vi "CRYInsert Data to Listbox Etc.vi"(4 "Type":enum16{"Curves", "Values", "Results", "WFM"}(ring)=enum."Results", 7 "sAction":string, 8 "Waveforms":T2[](array[typedef]) {"Y dB ref" format="%.1f"; "Y axis" items=["Log", "Lin"]; "Y data" items=["dB", "Lin"]; "X data" items=["dB", "Lin"]}, 9 "Results":T3[](array[typedef]) {"Margin" format="%.2f"}, 10 "Values":T1[](array[typedef]) {"Z data" items=["dB", "Lin"]; "X data" items=["dB", "Lin"]; "Y data" items=["dB", "Lin"]; "Z dB ref" format="%.1f"; "Z axis" items=["Log", "Lin"]; "X dB ref" format="%.1f"; "X axis" items=["Log", "Lin"]; "Y axis" items=["Log", "Lin"]; "Y dB ref" format="%.1f"; "Curve"."z" format="%.2f"; "Curve"."y" format="%.2f"; "Curve"."x" format="%.2f"}, 11 "Curves":T1[](array[typedef]) {"Z data" items=["dB", "Lin"]; "X data" items=["dB", "Lin"]; "Y data" items=["dB", "Lin"]; "Z dB ref" format="%.1f"; "Z axis" items=["Log", "Lin"]; "X dB ref" format="%.1f"; "X axis" items=["Log", "Lin"]; "Y axis" items=["Log", "Lin"]; "Y dB ref" format="%.1f"; "Curve"."z" format="%.2f"; "Curve"."y" format="%.2f"; "Curve"."x" format="%.2f"}) -> ()   [LabVIEW 2013]
uses:
  CRYSystem/Typedef Control/CRYData Cluster.ctl
  CRYSystem/Typedef Control/CRYResult Cluster.ctl
  CRYSystem/Typedef Control/CRYWaveform Cluster.ctl
  Global/CRYCurve Library Global.vi
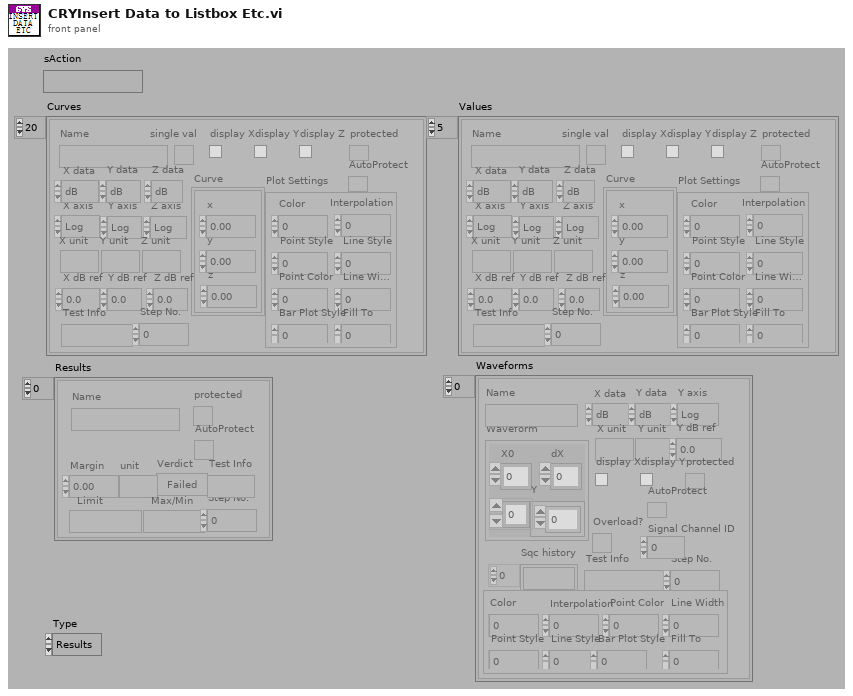
[diagram p1: front panel]
types:
  T1 = typedef "CRYData Cluster.ctl" = cluster{"Name":string, "Curve":cluster{"x":dbl, "y":dbl, "z":dbl}[], "X data":u16, "Y data":u16, "Z data":u16, "X axis":u16, "Y axis":u16, "Z axis":u16, "X unit":string, "Y unit":string, "Z unit":string, "X dB ref":dbl, "Y dB ref":dbl, "Z dB ref":dbl, "single val":bool, "protected":bool, "display X":bool, "display Y":bool, "display Z":bool, "Test Info":string, "Step No.":i32, "Plot Settings":cluster{"Color":u32, "Interpolation":u8, "Point Style":u8, "Line Style":u8, "Point Color":u32, "Line Width":u8, "Bar Plot Style":u8, "Fill To":i16}, "AutoProtect":bool}
  T2 = typedef "CRYWaveform Cluster.ctl" = cluster{"Waveform":cluster{"X0":dbl, "dX":dbl, "Y":sgl[]}, "X data":u16, "Y data":u16, "Y axis":u16, "X unit":string, "Y unit":string, "Y dB ref":dbl, "display Y":bool, "display X":bool, "Overload?":bool, "Test Info":string, "Step No.":i32, "Name":string, "protected":bool, "Sqc history":string[], "Signal Channel ID":i32, "Plot Settings":cluster{"Color":u32, "Interpolation":u8, "Point Style":u8, "Line Style":u8, "Point Color":u32, "Line Width":u8, "Bar Plot Style":u8, "Fill To":i16}, "AutoProtect":bool}
  T3 = typedef "CRYResult Cluster.ctl" = cluster{"Name":string, "Margin":dbl, "unit":string, "Verdict":bool, "Limit":string, "Max/Min":string, "protected":bool, "Step No.":i32, "Test Info":string, "AutoProtect":bool}
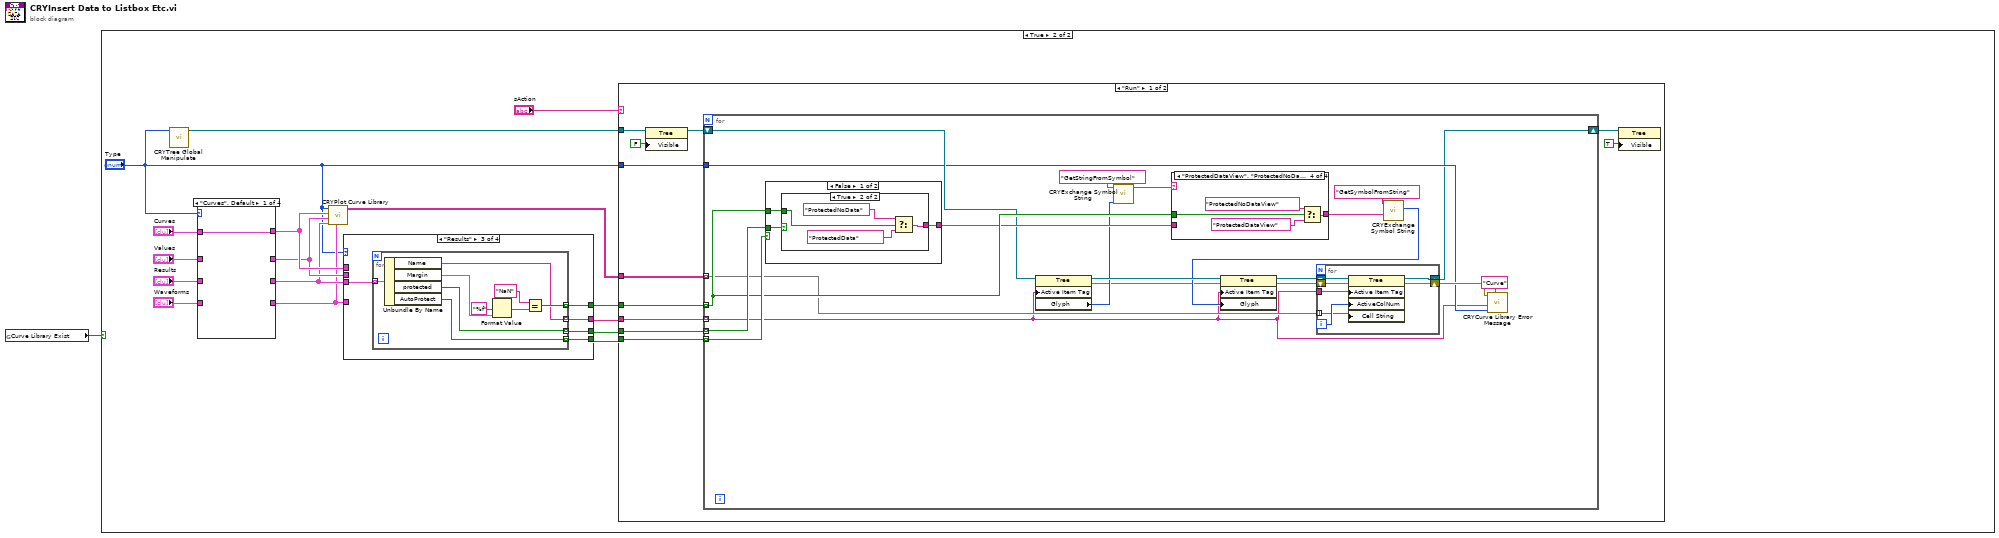
[diagram p0: block diagram]
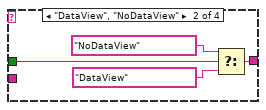
[diagram p4: hidden frame]
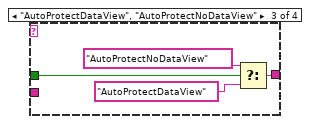
[diagram p5: hidden frame]
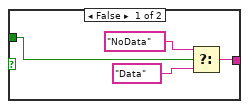
[diagram p6: hidden frame]
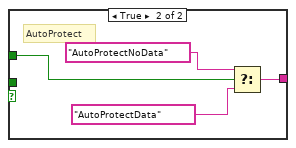
[diagram p7: hidden frame]
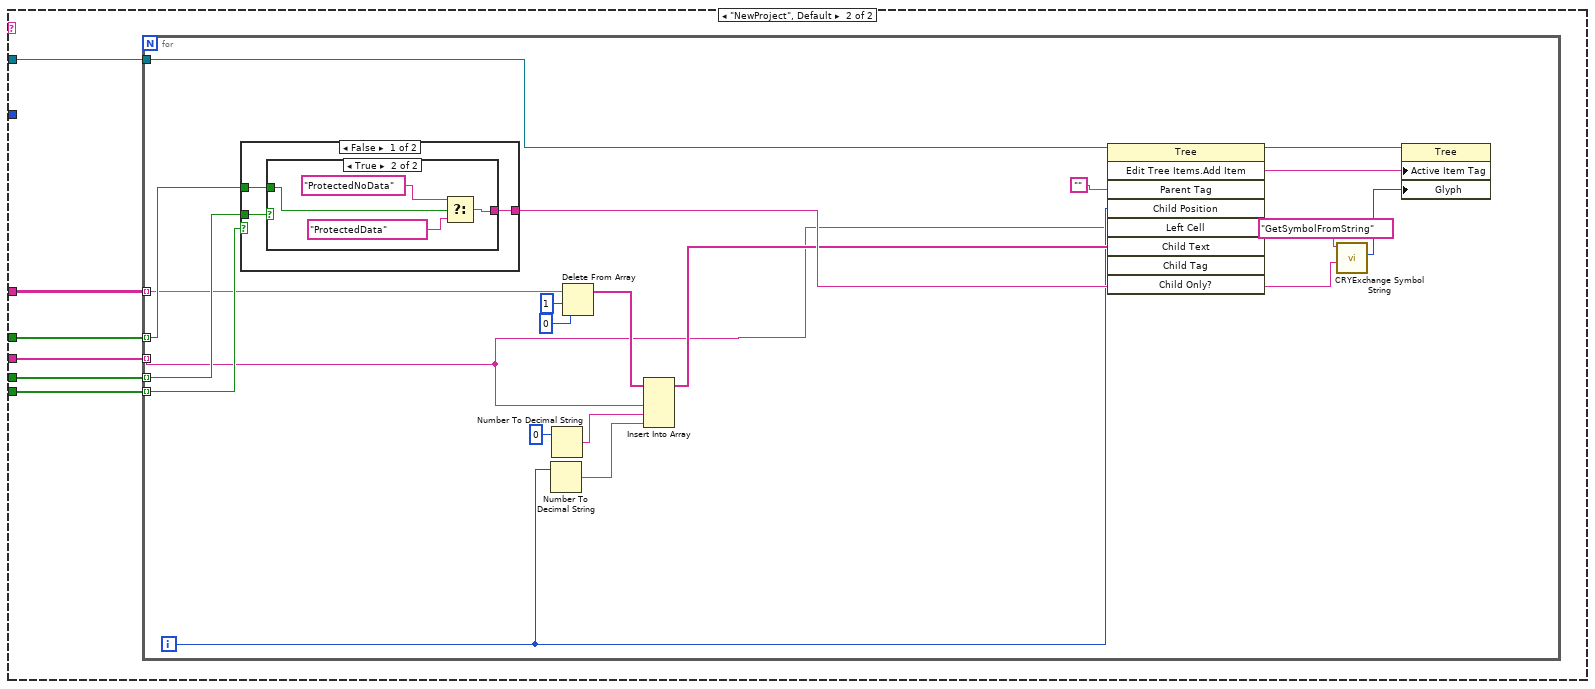
[diagram p8: hidden frame]
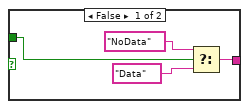
[diagram p9: hidden frame]
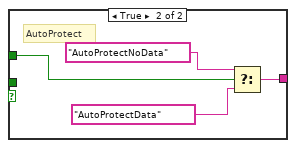
[diagram p10: hidden frame]
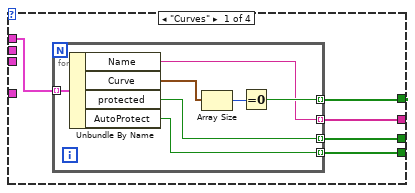
[diagram p11: hidden frame]
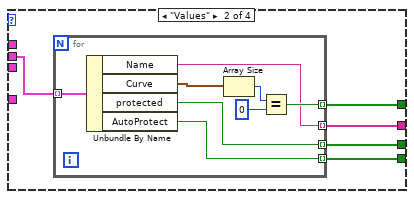
[diagram p12: hidden frame]
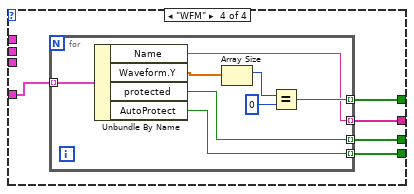
[diagram p13: hidden frame]
diagram:
  n1 = global read "CRYCurve Library Global.vi" "Curve Library Exist"() -> (w1:bool)
  n2 = case shown="True" w1 {
    frame False {
    }
    frame True {
      n3 = call "CRYTree Global Manipulate.vi"("Type In"="Type") -> ("Tree/Curve Tree"=w4:refnum<vi>)  [unwired: 7 in, 3 out]
      n4 = case shown="\"Curves\", Default" "Type" {
        tunnel: "Curves" -> [w178 _ _ _]
        tunnel: "Results" -> [_ _ w180 _]
        tunnel: [w178 _ _ _] -> w8
        tunnel: [_ _ w180 _] -> w6
        tunnel: "Waveforms" -> [_ _ _ w181]
        tunnel: [_ _ _ w181] -> w5
        tunnel: "Values" -> [_ w179 _ _]
        tunnel: [_ w179 _ _] -> w7
        frame "Curves", Default {
        }
        frame "Values" {
        }
        frame "Results" {
        }
        frame "WFM" {
        }
      }
      n5 = call "CRYPlot Curve Library.vi"("Waveform"=w5, "Results"=w6, "Values"=w7, "Curves"=w8, "Type"="Type") -> ("PlotStrings"=w13:string[][])  [unwired: 6 in]
      n6 = case shown="\"Results\"" "Type" {
        tunnel: [w130 w142 w155 w169] -> w17
        tunnel: [w129 w141 w154 w168] -> w16
        tunnel: [w128 w140 w153 w167] -> w15
        tunnel: [w127 w139 w152 w166] -> w14
        tunnel: w8 -> [w126 _ _ _]
        tunnel: w7 -> [_ w138 _ _]
        tunnel: w6 -> [_ _ w151 _]
        tunnel: w5 -> [_ _ _ w165]
        frame "Curves" {
          n7 = for {
            tunnel: w126 -> [w136] mode=indexing
            tunnel: [w135] -> w130 mode=indexing
            tunnel: [w131] -> w129 mode=indexing
            tunnel: [w133] -> w128 mode=indexing
            tunnel: [w132] -> w127 mode=indexing
            n8 = Unbundle By Name(w136) -> ("Name"=w131:string, "Curve"=w137:cluster{"x":dbl, "y":dbl, "z":dbl}[], "protected"=w133:bool, "AutoProtect"=w132:bool)
            n9 = Array Size(array=w137) -> (size(s)=w134:i32)
            n10 = Equal To 0?(x=w134) -> (x = 0?=w135:bool)
          }
        }
        frame "Values" {
          n11 = for {
            tunnel: w138 -> [w149] mode=indexing
            tunnel: [w146] -> w142 mode=indexing
            tunnel: [w143] -> w141 mode=indexing
            tunnel: [w145] -> w140 mode=indexing
            tunnel: [w144] -> w139 mode=indexing
            n12 = Unbundle By Name(w149) -> ("Name"=w143:string, "Curve"=w150:cluster{"x":dbl, "y":dbl, "z":dbl}[], "protected"=w145:bool, "AutoProtect"=w144:bool)
            n13 = Array Size(array=w150) -> (size(s)=w147:i32)
            n14 = Equal?(x=w147, y=0) -> (x = y?=w146:bool)
          }
        }
        frame "Results" {
          n15 = for {
            tunnel: w151 -> [w164] mode=indexing
            tunnel: [w163] -> w155 mode=indexing
            tunnel: [w156] -> w154 mode=indexing
            tunnel: [w158] -> w153 mode=indexing
            tunnel: [w157] -> w152 mode=indexing
            n16 = Unbundle By Name(w164) -> ("Name"=w156:string, "Margin"=w162:dbl, "protected"=w158:bool, "AutoProtect"=w157:bool)
            n17 = Format Value(format string="%f", value (0)=w162) -> (output string=w159:string)  [unwired: 1 in]
            n18 = Equal?(x="NaN", y=w159) -> (x = y?=w163:bool)
          }
        }
        frame "WFM" {
          n19 = for {
            tunnel: w165 -> [w174] mode=indexing
            tunnel: [w173] -> w169 mode=indexing
            tunnel: [w170] -> w168 mode=indexing
            tunnel: [w172] -> w167 mode=indexing
            tunnel: [w171] -> w166 mode=indexing
            n20 = Unbundle By Name(w174) -> ("Name"=w170:string, "Waveform.Y"=w176:sgl[], "protected"=w172:bool, "AutoProtect"=w171:bool)
            n21 = Array Size(array=w176) -> (size(s)=w177:i32)
            n22 = Equal?(x=w177, y=0) -> (x = y?=w173:bool)
          }
        }
      }
      n23 = case shown="\"Run\"" "sAction" {
        tunnel: w17 -> [w28 w90]
        tunnel: w16 -> [w27 w89]
        tunnel: w15 -> [w26 w88]
        tunnel: w14 -> [w25 w87]
        tunnel: w13 -> [w24 w86]
        tunnel: w4 -> [w22 w85]
        tunnel: "Type" -> [w23 _]
        frame "Run" {
          n24 = property class="Tree"(reference=w22, "Visible"=FALSE) -> (reference out=w20:refnum<vi>)  [unwired: 1 in, 1 out]
          n25 = for {
            tunnel: w24 -> [w46] mode=indexing
            tunnel: w28 -> [w47] mode=indexing
            tunnel: w27 -> [w31] mode=indexing
            tunnel: w26 -> [w48] mode=indexing
            tunnel: w25 -> [w49] mode=indexing
            tunnel: w23 -> [w32]
            shift-right: [w29] -> w18
            shift-left: w20 -> [w44]
            n26 = case shown="False" w49 {
              tunnel: w47 -> [w71 w84]
              tunnel: [w70 w83] -> w45
              tunnel: w48 -> [w72 _]
              frame False {
                n27 = case shown="True" w72 {
                  tunnel: w71 -> [w76 w80]
                  tunnel: [w75 w79] -> w70
                  frame False {
                    n28 = Select(t="NoData" ("name or relative path"), s=w76, f="Data" ("name or relative path")) -> (s? t:f=w75:string)
                  }
                  frame True {
                    n29 = Select(t="ProtectedNoData" ("name or relative path"), s=w80, f="ProtectedData" ("name or relative path")) -> (s? t:f=w79:string)
                  }
                }
              }
              frame True {
                # "AutoProtect"
                n30 = Select(t="AutoProtectNoData" ("name or relative path"), s=w84, f="AutoProtectData" ("name or relative path")) -> (s? t:f=w83:string)
              }
            }
            n31 = property on="Property Node" class="Tree"(reference=w44, "Active Item Tag"=w31) -> (reference out=w42:refnum<vi>, error out=w35:errorcluster, "Glyph"=w40:i32)  [unwired: 1 in]
            n32 = call "CRYExchange Symbol String.vi"("nData"=w40, "sAction"="GetStringFromSymbol") -> ("sData out"=w39:string)  [unwired: 8 in, 1 out]
            n33 = case shown="\"ProtectedDataView\", \"ProtectedNoDataView\"" w39 {
              tunnel: w47 -> [_ w61 w65 w69]
              tunnel: [w57 w60 w64 w68] -> w36
              tunnel: w45 -> [w57 _ _ _]
              frame Default {
              }
              frame "DataView", "NoDataView" {
                n34 = Select(t="NoDataView" ("name or relative path"), s=w61, f="DataView" ("name or relative path")) -> (s? t:f=w60:string)
              }
              frame "AutoProtectDataView", "AutoProtectNoDataView" {
                n35 = Select(t="AutoProtectNoDataView" ("name or relative path"), s=w65, f="AutoProtectDataView" ("name or relative path")) -> (s? t:f=w64:string)
              }
              frame "ProtectedDataView", "ProtectedNoDataView" {
                n36 = Select(t="ProtectedNoDataView" ("name or relative path"), s=w69, f="ProtectedDataView" ("name or relative path")) -> (s? t:f=w68:string)
              }
            }
            n37 = call "CRYExchange Symbol String.vi"("sData"=w36, "sAction"="GetSymbolFromString") -> ("nData out"=w37:i32)  [unwired: 8 in, 1 out]
            n38 = property on="Property Node" class="Tree"(reference=w42, error in=w35, "Active Item Tag"=w31, "Glyph"=w37) -> (reference out=w43:refnum<vi>, error out=w34:errorcluster)
            n39 = for {
              shift-right: [w55] -> w29
              shift-left: w43 -> [w56]
              tunnel: w31 -> [w54]
              tunnel: w46 -> [w52] mode=indexing
              shift-right: [w50] -> w33
              shift-left: w34 -> [w51]
              i -> [w53]
              n40 = property on="Property Node" class="Tree"(reference=w56, error in=w51, "Active Item Tag"=w54, "ActiveColNum"=w53, "Cell String"=w52) -> (reference out=w55:refnum<vi>, error out=w50:errorcluster)
            }
            n41 = call "CRYCurve Library Error Message.vi"("sAction"="Curve", "Type"=w32, "sData"=w31, "error IO"=w33) -> ()  [unwired: 8 in]
          }
          n42 = property class="Tree"(reference=w18, "Visible"=TRUE) -> ()  [unwired: 1 in, 2 out]
        }
        frame "NewProject", Default {
          n43 = for {
            tunnel: w86 -> [w105] mode=indexing
            tunnel: w90 -> [w108] mode=indexing
            tunnel: w89 -> [w93] mode=indexing
            tunnel: w88 -> [w109] mode=indexing
            tunnel: w87 -> [w110] mode=indexing
            tunnel: w85 -> [w100]
            i -> [w94]
            n44 = case shown="False" w110 {
              tunnel: w108 -> [w112 w125]
              tunnel: [w111 w124] -> w104
              tunnel: w109 -> [w113 _]
              frame False {
                n45 = case shown="True" w113 {
                  tunnel: w112 -> [w117 w121]
                  tunnel: [w116 w120] -> w111
                  frame False {
                    n46 = Select(t="NoData" ("name or relative path"), s=w117, f="Data" ("name or relative path")) -> (s? t:f=w116:string)
                  }
                  frame True {
                    n47 = Select(t="ProtectedNoData" ("name or relative path"), s=w121, f="ProtectedData" ("name or relative path")) -> (s? t:f=w120:string)
                  }
                }
              }
              frame True {
                # "AutoProtect"
                n48 = Select(t="AutoProtectNoData" ("name or relative path"), s=w125, f="AutoProtectData" ("name or relative path")) -> (s? t:f=w124:string)
              }
            }
            n49 = Number To Decimal String(number=w94) -> (decimal integer string=w103:string)  [unwired: 1 in]
            n50 = Number To Decimal String(number=0) -> (decimal integer string=w92:string)  [unwired: 1 in]
            n51 = Delete From Array(array=w105, length=1, index=0) -> (array with subset deleted=w102:string[])  [unwired: 1 out]
            n52 = Insert Into Array(array=w102, new element #1=w93, new element #2=w92, new element #3=w103) -> (w101:string[])  [unwired: 1 in]
            n53 = invoke class="Tree" method="Edit Tree Items.Add Item"(reference=w100, "Parent Tag"="", "Child Position"=w94, "Left Cell"=w93, "Child Text"=w101) -> (reference out=w98:refnum<vi>, "Edit Tree Items:Add Item"=w99:string)  [unwired: 4 in, 7 out]
            n54 = call "CRYExchange Symbol String.vi"("sData"=w104, "sAction"="GetSymbolFromString") -> ("nData out"=w96:i32)  [unwired: 8 in, 1 out]
            n55 = property class="Tree"(reference=w98, "Active Item Tag"=w99, "Glyph"=w96) -> ()  [unwired: 1 in, 2 out]
          }
        }
      }
    }
  }
